vi "Execute.vi"(8 "error in (no error)":errorcluster, 10 "System In":refnum<class "bt_System.lvclass">, 11 "Node in":refnum<class "bt_Blackboard Boolean Set.lvclass">) -> (0 "error out":errorcluster, 1 "Status":T1, 2 "System Out":refnum<class "bt_System.lvclass">, 3 "Node out":refnum<class "bt_Blackboard Boolean Set.lvclass">)   [LabVIEW 2021, in "BT.lvlib" / "bt_Blackboard Boolean Set.lvclass"]
uses:
  bt_Blackboard Boolean Set.lvclass
  C:/Users/Tim/Documents/GitHub/LV_Behaviour_Tree/Source/Support/Nodes/Leaves/Blackboard/Type/bt_Blackboard_Leaf Type.lvclass
  Support/Nodes/abs_Node/Status.ctl
  Support/abs_System/bt_System.lvclass
  Support/Nodes/Leaves/Blackboard/Type/bt_Blackboard_Leaf Type.lvclass/bt_Blackboard_Leaf Type.ctl
  bt_Blackboard Boolean Set.lvclass/bt_Blackboard Boolean Set.ctl
  Support/abs_System/bt_System.lvclass/bt_System.ctl
  Support/Blackboard/bt_Blackboard.lvclass/bt_Blackboard.ctl
  Support/Nodes/Leaves/Blackboard/Type/Properties/Read Group Index.vi
  Support/Nodes/Leaves/Blackboard/Type/Properties/Read Tag Index.vi
  Properties/Read Value.vi
  Support/abs_System/Properties/Read Blackboard.vi
  Support/Blackboard/Properties/Read Data.vi
  Support/Blackboard/Properties/Write Data.vi
  Support/abs_System/Properties/Write Blackboard.vi
  Support/Blackboard/bt_Blackboard.lvclass
  Support/Nodes/abs_Node/bt_Node.lvclass
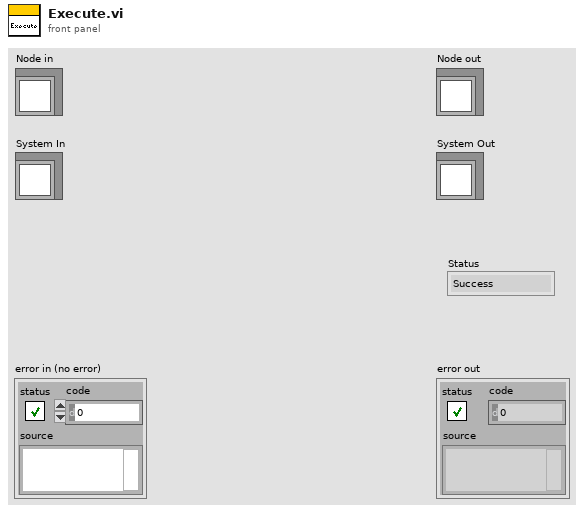
[diagram p1: front panel]
types:
  T1 = typedef "BT.lvlib/bt_Node.lvclass/Status.ctl" = enum16{"Success", "Failure", "Running"}
  T2 = typedef "BT.lvlib/bt_Blackboard.lvclass/Data DVR Type.ctl" = cluster{"Boolean":cluster{"Tags":refnum<data-value>, "Boolean":refnum<data-value>, "Status":refnum<data-value>}, "String":cluster{"Tags":refnum<data-value>, "String":refnum<data-value>, "Status":refnum<data-value>}, "DBL":cluster{"Tags":refnum<data-value>, "DBL":refnum<data-value>, "Status":refnum<data-value>}, "SGL":cluster{"Tags":refnum<data-value>, "SGL":refnum<data-value>, "Status":refnum<data-value>}, "EXT":cluster{"Tags":refnum<data-value>, "EXT":refnum<data-value>, "Status":refnum<data-value>}, "U8":cluster{"Tags":refnum<data-value>, "U8":refnum<data-value>, "Status":refnum<data-value>}, "U16":cluster{"Tags":refnum<data-value>, "U16":refnum<data-value>, "Status":refnum<data-value>}, "U32":cluster{"Tags":refnum<data-value>, "U32":refnum<data-value>, "Status":refnum<data-value>}, "U64":cluster{"Tags":refnum<data-value>, "U64":refnum<data-value>, "Status":refnum<data-value>}, "I8":cluster{"Tags":refnum<data-value>, "I8":refnum<data-value>, "Status":refnum<data-value>}, "I16":cluster{"Tags":refnum<data-value>, "I16":refnum<data-value>, "Status":refnum<data-value>}, "I32":cluster{"Tags":refnum<data-value>, "I32":refnum<data-value>, "Status":refnum<data-value>}, "I64":cluster{"Tags":refnum<data-value>, "I64":refnum<data-value>, "Status":refnum<data-value>}, "CDBL":cluster{"Tags":refnum<data-value>, "CDBL":refnum<data-value>, "Status":refnum<data-value>}, "CSGL":cluster{"Tags":refnum<data-value>, "CSGL":refnum<data-value>, "Status":refnum<data-value>}, "CEXT":cluster{"Tags":refnum<data-value>, "CEXT":refnum<data-value>, "Status":refnum<data-value>}, "Time":cluster{"Tags":refnum<data-value>, "Time":refnum<data-value>, "Status":refnum<data-value>}, "Variant":cluster{"Tags":refnum<data-value>, "Variant":refnum<data-value>, "Status":refnum<data-value>}, "Waveform":cluster{"Tags":refnum<data-value>, "Waveform":refnum<data-value>, "Status":refnum<data-value>}}
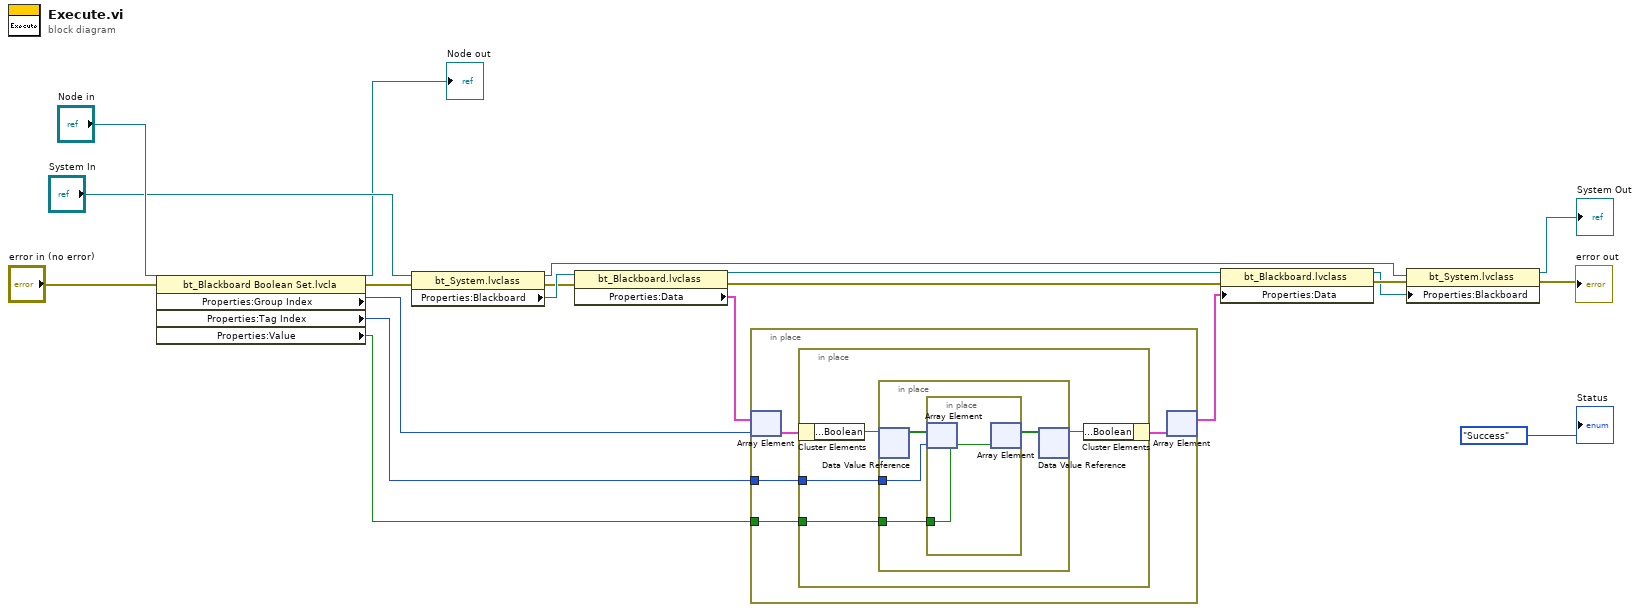
[diagram p0: block diagram]
diagram:
  n1 = property class="bt_Blackboard Boolean Set.lvcla"(reference="Node in", error in="error in (no error)") -> (reference out=→"Node out":refnum<class "bt_Blackboard Boolean Set.lvclass">, error out=w18:errorcluster, "Properties:Group Index"=w12:i32, "Properties:Tag Index"=w2:i32, "Properties:Value"=w1:bool)
  n2 = property class="bt_System.lvclass"(reference="System In", error in=w18) -> (reference out=w5:refnum<class "bt_System.lvclass">, error out=w14:errorcluster, "Properties:Blackboard"=w15:refnum<class "bt_Blackboard.lvclass">)
  n3 = property class="bt_Blackboard.lvclass"(reference=w15, error in=w14) -> (reference out=w9:refnum<class "bt_Blackboard.lvclass">, error out=w10:errorcluster, "Properties:Data"=w13:T2[])
  n4 = in-place {
    in-place-border: w2 -> [w23]
    in-place-border: w1 -> [w22]
    n5 = in-place-array #1(w13, w12) -> (w24:T2)
    n6 = in-place {
      in-place-border: w23 -> [w26]
      in-place-border: w22 -> [w25]
      n7 = in-place-cluster #2(w24) -> ("Boolean.Boolean"=w28:refnum<data-value>)
      n8 = in-place {
        in-place-border: w26 -> [w30]
        in-place-border: w25 -> [w29]
        n9 = in-place-dvr #3(w28) -> (w32:bool[])  [unwired: 1 out]
        n10 = in-place {
          in-place-border: w29 -> [w33]
          n11 = in-place-array #4(w32, w30) -> ()  [unwired: 1 out]
          n12 = in-place-array #4(w33) -> (w31:bool[])  [unwired: 1 out]
        }
        n13 = in-place-dvr #3(w31) -> (w27:refnum<data-value>)  [unwired: 1 out]
      }
      n14 = in-place-cluster #2("Boolean.Boolean"=w27) -> (w21:T2)
    }
    n15 = in-place-array #1(w21) -> (w8:T2[])  [unwired: 1 out]
  }
  n16 = property class="bt_Blackboard.lvclass"(reference=w9, error in=w10, "Properties:Data"=w8) -> (reference out=w6:refnum<class "bt_Blackboard.lvclass">, error out=w7:errorcluster)
  n17 = property class="bt_System.lvclass"(reference=w5, error in=w7, "Properties:Blackboard"=w6) -> (reference out=→"System Out":refnum<class "bt_System.lvclass">, error out=→"error out":errorcluster)
  "Status" <- Status."Success" ("Status")
